vi "PID Drive.vi"(8 "Targets":T2, 9 "Tolerances":T3, 10 "Motor Values":T4, 11 "Drive PID Gains":T1) -> (1 "Y Out":dbl, 2 "X Out":dbl, 3 "Finished?":bool)   [LabVIEW 2017]
uses:
  Common Code/PID Gains Cluster.ctl
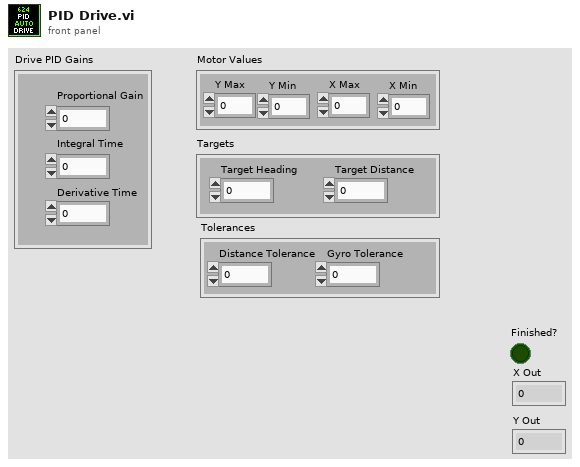
[diagram p1: front panel]
types:
  T1 = typedef "PID Gains Cluster.ctl" = cluster{"Integral Time":dbl, "Proportional Gain":dbl, "Derivative Time":dbl}
  T2 = cluster{"Target Heading":dbl, "Target Distance":dbl}
  T3 = cluster{"Distance Tolerance":dbl, "Gyro Tolerance":dbl}
  T4 = cluster{"Y Max":dbl, "Y Min":dbl, "X Min":dbl, "X Max":dbl}
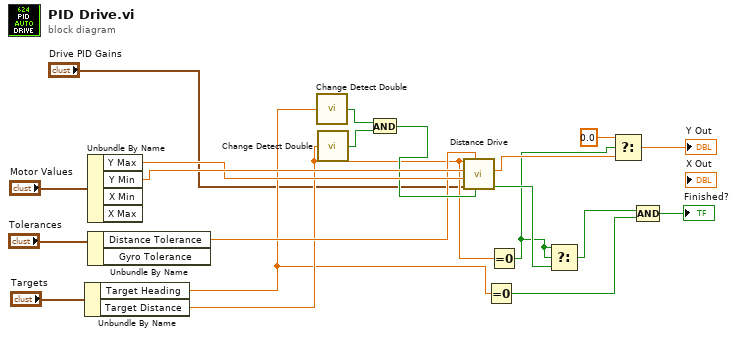
[diagram p0: block diagram]
diagram:
  n1 = Unbundle By Name("Targets") -> ("Target Heading"=w3:dbl, "Target Distance"=w7:dbl)
  n2 = Unbundle By Name("Motor Values") -> ("Y Max"=w14:dbl, "Y Min"=w15:dbl)  [unwired: 2 out]
  n3 = Unbundle By Name("Tolerances") -> ("Distance Tolerance"=w12:dbl)  [unwired: 1 out]
  n4 = call "Change Detect Double.vi"("In"=w3) -> ("Changed?"=w17:bool)
  n5 = call "Change Detect Double.vi"("In"=w7) -> ("Changed?"=w16:bool)
  n6 = And(x=w17, y=w16) -> (x .and. y?=w13:bool)
  n7 = call "Distance Drive.vi"("ReInit?"=w13, "Distance Tolerance"=w12, "PID Gains"="Drive PID Gains", "Y Max Output"=w14, "Y Min Output"=w15, "Distance Target"=w7) -> ("Finished"=w6:bool, "Y Output"=w10:dbl)  [unwired: 4 in]
  n8 = Equal To 0?(x=w3) -> (x = 0?=w1:bool)
  n9 = Equal To 0?(x=w7) -> (x = 0?=w5:bool)
  n10 = Select(t=w5, s=w5, f=w6) -> (s? t:f=w4:bool)
  n11 = Select(t=0.0, s=w5, f=w10) -> (s? t:f=→"Y Out":dbl)
  n12 = Compound Arithmetic op=AND(w4, w1) -> (→"Finished?":bool)
